vi "CPP_GaussianPlume.vi"() -> (5 "Plug in titles":string[](array[string]), 7 "Plug in values":string[](array[string]))   [LabVIEW 2011]
uses:
  Globals/Meas_global.vi
  Utilities/gaussianFit/GaussianGlobal.vi
panel:
  out "FitSDwithin(Factor)OfPrediction?":bool
  out "bigEnough?":bool
  out "closeEnough?":bool
  in  "AmplitudeTolerance (%)":dbl=5.0
  in  "LocationTolerance":dbl=0.1 caption="LocationTolerance(*predictedSD)"
  in  "FitvsPredictionSDFactor":dbl=2.0
  out "ConcentrationData":dbl[](array[numeric])
  out "PositionData":dbl[](array[numeric])
  out "FitStatus":string
  out "FitResidual":dbl
  out "FitStdDev":dbl
  out "FitMax":dbl
  out "FitCenter":dbl
  out "XY Graph":T1(graph)
  # "!! 5-hole 1-5 must be connected to Channels 1-5 !!"
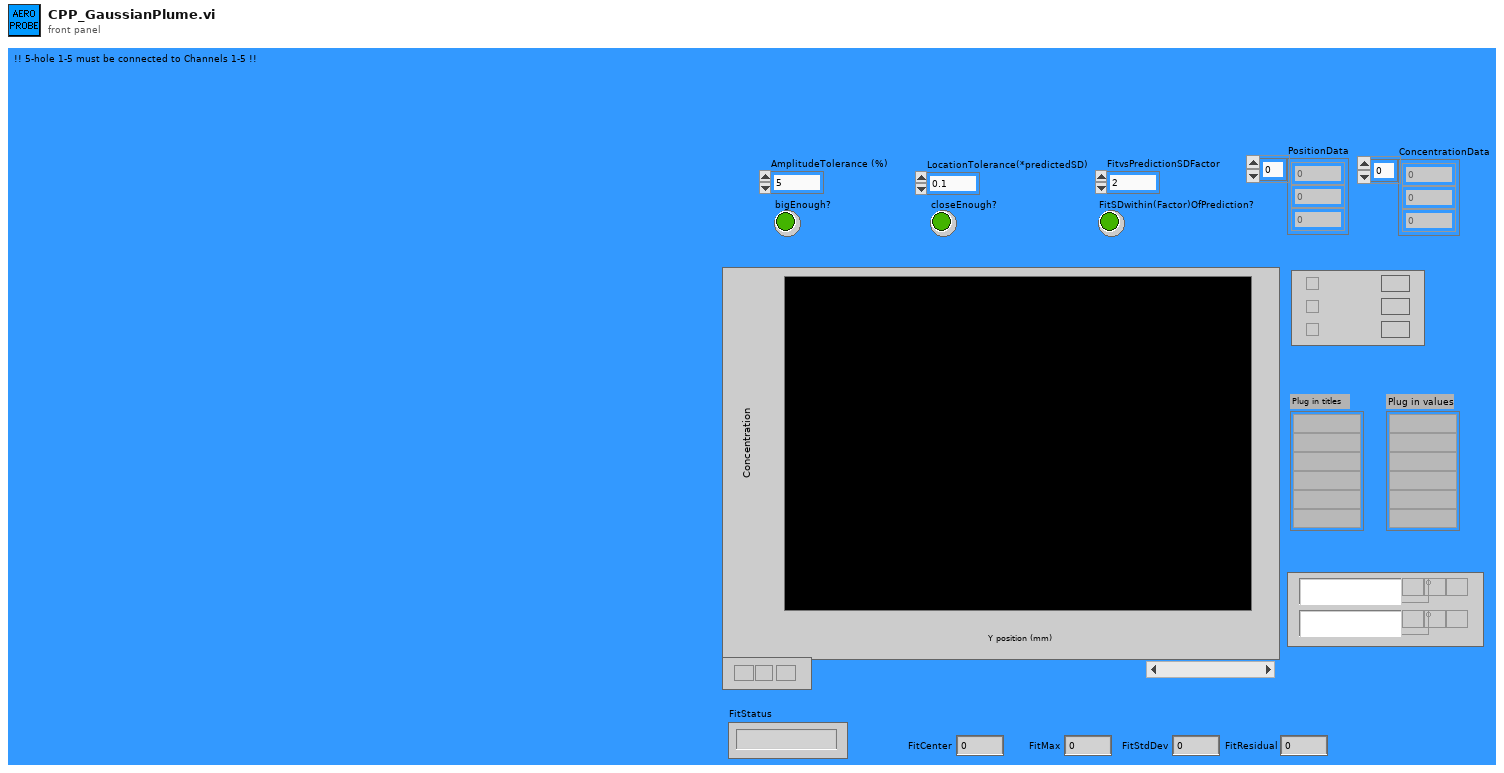
[diagram p1: front panel]
types:
  T1 = cluster{"Array - Numeric":dbl[], "Array - Numeric":dbl[]}[]
  T2 = typedef "Analysis_info_cluster.ctl" = cluster{"Colour":u32, "Inst type":T3, "Inst name":string, "Symbol":string, "Code name":string, "Extra Info":string, "Inst Array":T4, "Extra Titles":string[], "Extra Values":string[], "Eng Values":dbl[], "Time (ms)":dbl[], "Voltage":dbl[], "U":dbl, "u^2":dbl, "u^3":dbl, "u^4":dbl, "Skew_u":dbl, "Kurt_u":dbl, "Sd Error in Mean":dbl, "% u'/U":dbl, "X":dbl, "Y":dbl, "Z":dbl, "Spectra":T5, "Autocorrelation":T5, "Timescale integral to 25%":dbl, "Sd Error in Variance":dbl, "Calib File":path, "Calib Constants":dbl[], "Histogram":T5, "Output Position":bool, "Full Stats":bool, "Weighting":dbl[], "Av Sampling Rate":dbl, "Av No of Samples":dbl, "Total Meas Time (s)":dbl}
  T3 = typedef "Inst_type.ctl" = enum16{"Propeller anemometer", "Raw voltage", "Pressure Transducer", "Pitot-static tube", "Preston tube", "Hot wire", "Cross wire 1", "Cross wire 2", "Generic Linear", "Generic Polynomial", "Generic BackPoly", "Fast FID", "Thermocouple", "Cold wire", "Pulsed Wire", "LDA Vel", "LDA Tran time", "LDA Arr time"}
  T4 = typedef "Instrument_Array.ctl" = enum16{"PWA", "LDA", "Analogue"}
  T5 = typedef "XY_Plot_Cluster.ctl" = cluster{"First Name":string, "Second Name":string, "X axis name":string, "Y axis name":string, "X array":dbl[], "Y array":dbl[]}
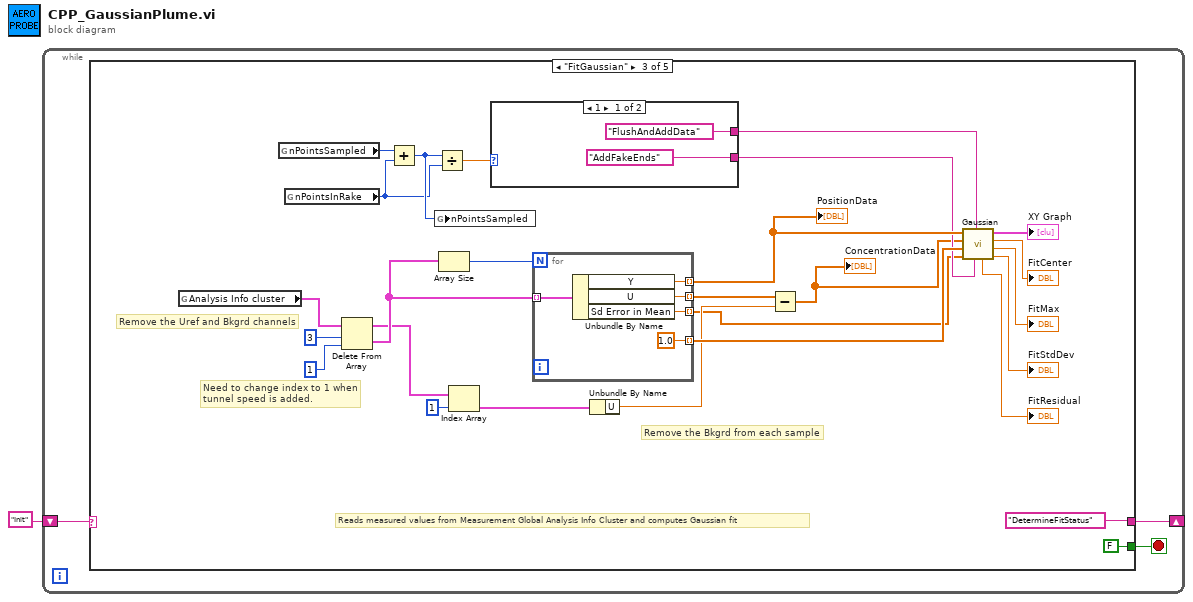
[diagram p0: block diagram]
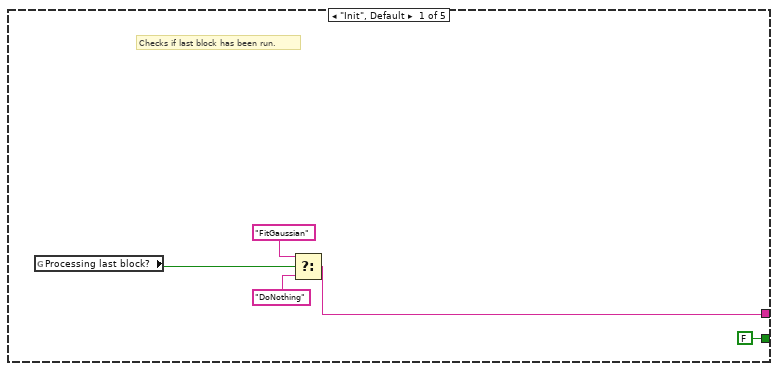
[diagram p2: hidden frame]
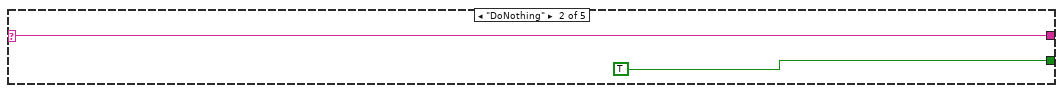
[diagram p3: hidden frame]
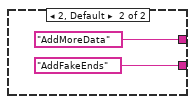
[diagram p4: hidden frame]
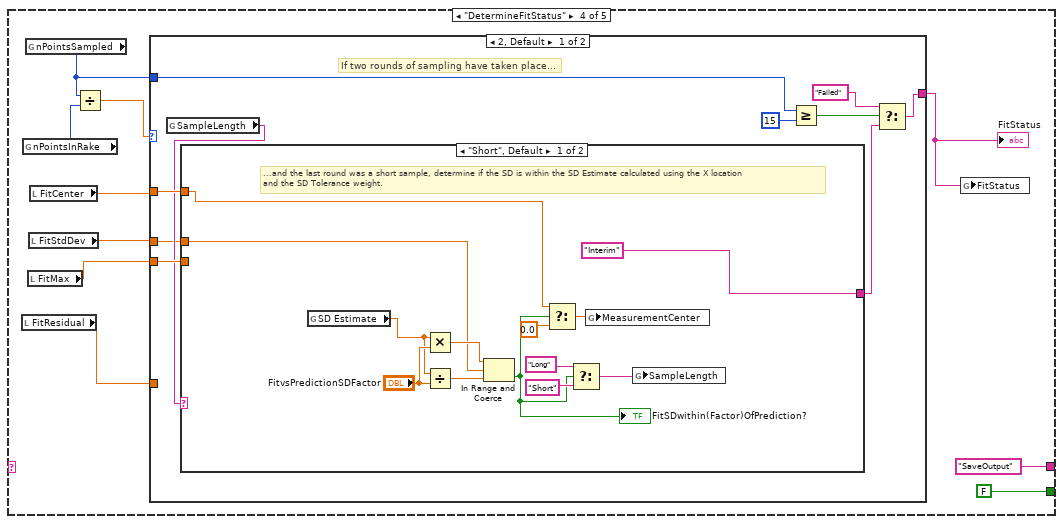
[diagram p5: hidden frame]
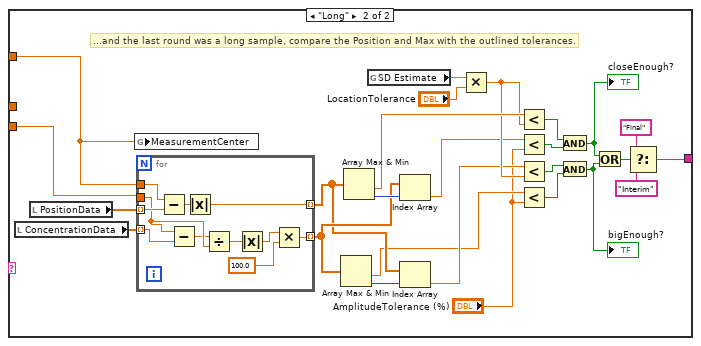
[diagram p6: hidden frame]
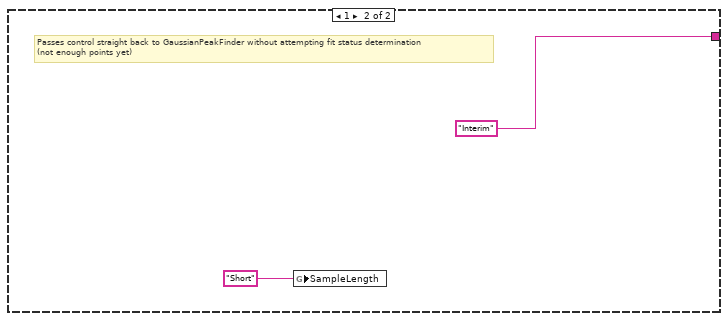
[diagram p7: hidden frame]
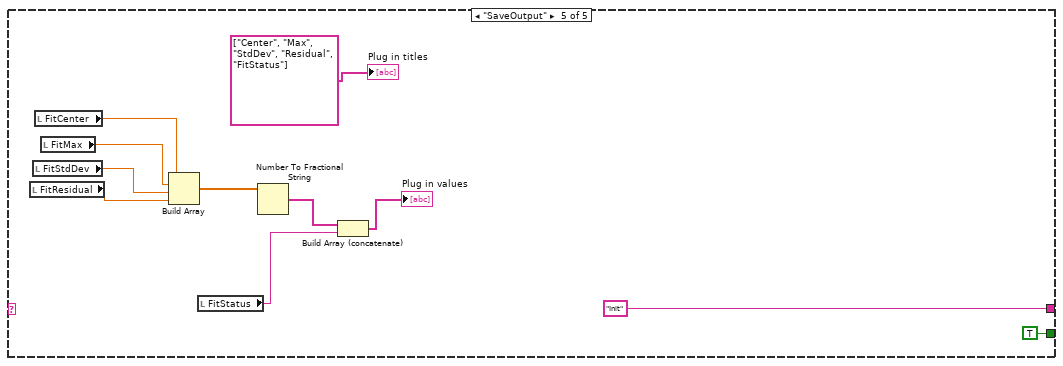
[diagram p8: hidden frame]
diagram:
  n1 = while {
    shift-right: [w3] -> _
    shift-left: "Init" -> [w4]
    stop <- w2 stop-if-true
    n2 = case shown="\"FitGaussian\"" w4 {
      selector: w4 -> [_ w11 _ _ _]
      tunnel: [w9 w11 "DetermineFitStatus" ("f") "SaveOutput" "Init"] -> w3
      tunnel: [FALSE TRUE FALSE FALSE TRUE] -> w2
      frame "Init", Default {
        # "Checks if last block has been run."
        n3 = global read "Meas_global.vi" "Processing last block?"() -> (w8:bool)
        n4 = Select(t="FitGaussian", s=w8, f="DoNothing") -> (s? t:f=w9:string)
      }
      frame "DoNothing" {
      }
      frame "FitGaussian" {
        # "Need to change index to 1 when\ntunnel speed is added."
        # "Remove the Bkgrd from each sample"
        # "Remove the Uref and Bkgrd channels"
        # "Reads measured values from Measurement Global Analysis Info Cluster and computes Gaussian fit"
        n5 = global read "Meas_global.vi" "Analysis Info cluster"() -> (w23:T2[])
        n6 = global read "GaussianGlobal.vi" "nPointsSampled"() -> (w27:i32)
        n7 = global read "GaussianGlobal.vi" "nPointsInRake"() -> (w25:i32)
        n8 = Delete From Array(array=w23, length=3, index=1) -> (deleted portion=w20:T2[], array with subset deleted=w19:T2[])
        n9 = Add(x=w27, y=w25) -> (x+y=w26:i32)
        n10 = global write "GaussianGlobal.vi" "nPointsSampled"(w26) -> ()
        n11 = Divide(x=w26, y=w25) -> (x/y=w30:dbl)
        n12 = Array Size(array=w20) -> (size(s)=w21:i32)
        n13 = Index Array(array=w19, index=1) -> (element=w18:T2)
        n14 = case shown="1" w30 {
          tunnel: ["FlushAndAddData" ("Mode") "AddMoreData" ("Mode")] -> w29
          tunnel: ["AddFakeEnds" ("Combo Box") "AddFakeEnds" ("Combo Box")] -> w28
          frame 1 {
          }
          frame 2, Default {
          }
        }
        n15 = for {
          N: w21 -> [_]
          tunnel: w20 -> [w43] mode=indexing
          tunnel: [w47] -> w38 mode=indexing
          tunnel: [w46] -> w13 mode=indexing
          tunnel: [w45] -> w12 mode=indexing
          tunnel: [1.0] -> w37 mode=indexing
          n16 = Unbundle By Name(w43) -> ("Y"=w47:dbl, "U"=w46:dbl, "Sd Error in Mean"=w45:dbl)
        }
        "PositionData" <- w38
        n17 = Unbundle By Name(w18) -> ("U"=w17:dbl)
        n18 = Subtract(x=w13, y=w17) -> (x-y=w16:dbl[])
        "ConcentrationData" <- w16
        n19 = call "Gaussian.vi"("Fake Ends?"=w28, "Mode"=w29, "YerrorIn"=w12, "XerrorIn"=w37, "YdataIn"=w16, "XdataIn"=w38) -> ("StdDev"=→"FitStdDev":dbl, "Max"=→"FitMax":dbl, "Center"=→"FitCenter":dbl, "XY Graph"=→"XY Graph":T1, "residual"=→"FitResidual":dbl)  [unwired: 1 in]
      }
      frame "DetermineFitStatus" {
        n20 = local read "FitResidual"() -> (w51:dbl)
        n21 = global read "GaussianGlobal.vi" "nPointsInRake"() -> (w56:i32)
        n22 = global read "GaussianGlobal.vi" "nPointsSampled"() -> (w48:i32)
        n23 = local read "FitMax"() -> (w53:dbl)
        n24 = local read "FitStdDev"() -> (w54:dbl)
        n25 = local read "FitCenter"() -> (w52:dbl)
        n26 = Divide(x=w48, y=w56) -> (x/y=w55:dbl)
        n27 = case shown="2, Default" w55 {
          tunnel: w54 -> [w58 _]
          tunnel: w53 -> [w66 _]
          tunnel: w52 -> [w67 _]
          tunnel: w51 -> [_ _]
          tunnel: [w60 "Interim"] -> w49
          tunnel: w48 -> [w64 _]
          frame 2, Default {
            # "If two rounds of sampling have taken place..."
            n28 = global read "GaussianGlobal.vi" "SampleLength"() -> (w65:string)
            n29 = case shown="\"Short\", Default" w65 {
              tunnel: w67 -> [w70 w81]
              tunnel: w66 -> [_ w106]
              tunnel: ["Interim" w83] -> w61
              tunnel: w58 -> [w68 _]
              frame "Short", Default {
                # "...and the last round was a short sample, determine if the SD is within the SD Estimate calculated using the X location\nand the SD Tolerance weight."
                n30 = global read "GaussianGlobal.vi" "SD Estimate"() -> (w78:dbl)
                n31 = Multiply(x=w78, y="FitvsPredictionSDFactor") -> (x*y=w80:dbl)
                n32 = Divide(x=w78, y="FitvsPredictionSDFactor") -> (x/y=w77:dbl)
                n33 = In Range and Coerce(upper limit=w80, x=w68, lower limit=w77) -> (In Range?=w73:bool)  [unwired: 1 out]
                "FitSDwithin(Factor)OfPrediction?" <- w73
                n34 = Select(t=w70, s=w73, f=0.0) -> (s? t:f=w72:dbl)
                n35 = Select(t="Long", s=w73, f="Short") -> (s? t:f=w74:string)
                n36 = global write "GaussianGlobal.vi" "MeasurementCenter"(w72) -> ()
                n37 = global write "GaussianGlobal.vi" "SampleLength"(w74) -> ()
              }
              frame "Long" {
                # "...and the last round was a long sample, compare the Position and Max with the outlined tolerances."
                n38 = local read "ConcentrationData"() -> (w105:dbl[])
                n39 = local read "PositionData"() -> (w104:dbl[])
                n40 = global write "GaussianGlobal.vi" "MeasurementCenter"(w81) -> ()
                n41 = for {
                  tunnel: w104 -> [w117] mode=indexing
                  tunnel: w105 -> [w116] mode=indexing
                  tunnel: w81 -> [w115]
                  tunnel: w106 -> [w114]
                  tunnel: [w109] -> w102 mode=indexing
                  tunnel: [w107] -> w100 mode=indexing
                  n42 = Subtract(x=w115, y=w117) -> (x-y=w108:dbl)
                  n43 = Subtract(x=w114, y=w116) -> (x-y=w113:dbl)
                  n44 = Absolute Value(x=w108) -> (abs(x)=w107:dbl)
                  n45 = Divide(x=w113, y=w114) -> (x/y=w112:dbl)
                  n46 = Absolute Value(x=w112) -> (abs(x)=w110:dbl)
                  n47 = Multiply(x=w110, y=100.0) -> (x*y=w109:dbl)
                }
                n48 = Array Max & Min(array=w102) -> (min value=w93:dbl, min index (indices)=w101:i32)  [unwired: 2 out]
                n49 = Array Max & Min(array=w100) -> (min value=w99:dbl, min index (indices)=w103:i32)  [unwired: 2 out]
                n50 = global read "GaussianGlobal.vi" "SD Estimate"() -> (w97:dbl)
                n51 = Index Array(array=w102, index=w103) -> (element=w95:dbl)
                n52 = Index Array(array=w100, index=w101) -> (element=w94:dbl)
                n53 = Multiply(x=w97, y="LocationTolerance") -> (x*y=w96:dbl)
                n54 = Less?(x=w99, y=w96) -> (x < y?=w91:bool)
                n55 = Less?(x=w95, y="AmplitudeTolerance (%)") -> (x < y?=w90:bool)
                n56 = Less?(x=w94, y=w96) -> (x < y?=w89:bool)
                n57 = Less?(x=w93, y="AmplitudeTolerance (%)") -> (x < y?=w88:bool)
                n58 = And(x=w91, y=w90) -> (x .and. y?=w87:bool)
                "closeEnough?" <- w87
                n59 = And(x=w89, y=w88) -> (x .and. y?=w86:bool)
                "bigEnough?" <- w86
                n60 = Or(x=w87, y=w86) -> (x .or. y?=w84:bool)
                n61 = Select(t="Final", s=w84, f="Interim") -> (s? t:f=w83:string)
              }
            }
            n62 = Greater Or Equal?(x=w64, y=15) -> (x >= y?=w62:bool)
            n63 = Select(t="Failed", s=w62, f=w61) -> (s? t:f=w60:string)
          }
          frame 1 {
            # "Passes control straight back to GaussianPeakFinder without attempting fit status determination\n(not enough points yet)"
            n64 = global write "GaussianGlobal.vi" "SampleLength"("Short" ("SampleLength")) -> ()
          }
        }
        "FitStatus" <- w49
        n65 = global write "GaussianGlobal.vi" "FitStatus"(w49) -> ()
      }
      frame "SaveOutput" {
        (unwired) TRUE
        n66 = local read "FitResidual"() -> (w125:dbl)
        n67 = local read "FitStdDev"() -> (w126:dbl)
        n68 = local read "FitCenter"() -> (w128:dbl)
        n69 = local read "FitMax"() -> (w127:dbl)
        n70 = Build Array(w128, w127, w126, w125) -> (w124:dbl[])
        n71 = local read "FitStatus"() -> (w122:string)
        n72 = Number To Fractional String(number=w124) -> (F-format string=w123:string[])  [unwired: 3 in]
        n73 = Build Array (concatenate)(w123, w122) -> (→"Plug in values":string[])
        "Plug in titles" <- string[] ["Center", "Max", "StdDev", "Residual", "FitStatus"] ("Plug in titles")
      }
    }
  }
